vi "Main.vi"() -> ()   [LabVIEW 2018]
uses:
  ctl/State.ctl
panel:
  out "시간계산":i32
  out "조리 시간":string
  in  "10초":bool
  in  "30초":bool
  in  "1분":bool
  in  "정지":bool
  out "출력 메세지":string
  in  "문 열림":bool
  in  "조리 시작":bool
  # "전자레인지"
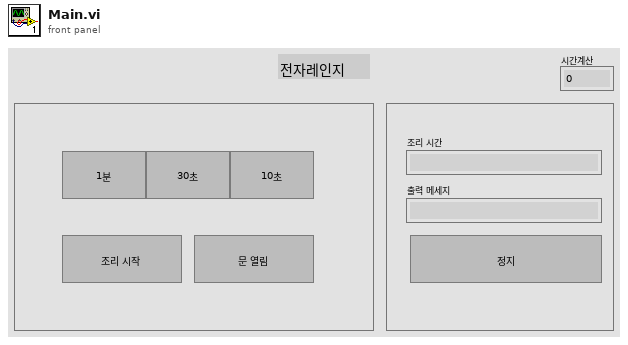
[diagram p1: front panel]
types:
  T1 = typedef "State.ctl" = enum16{"대기", "조리", "문열림", "조리완료", "일시정지"}
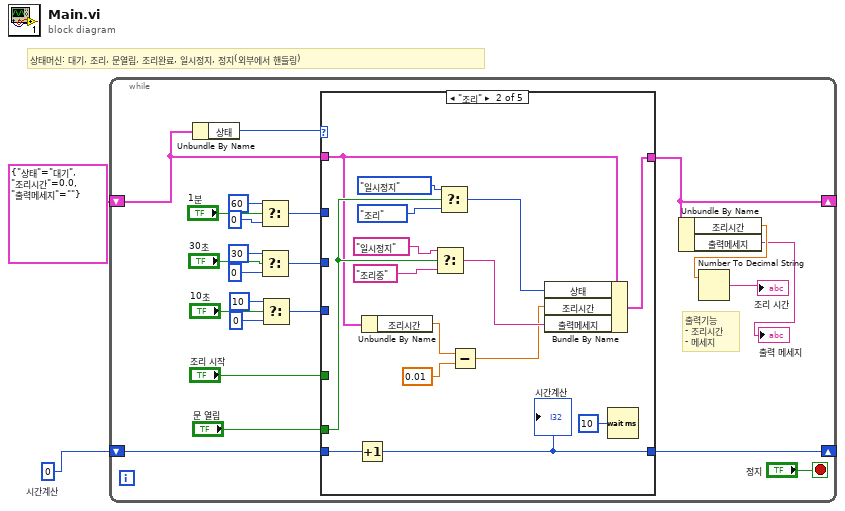
[diagram p0: block diagram]
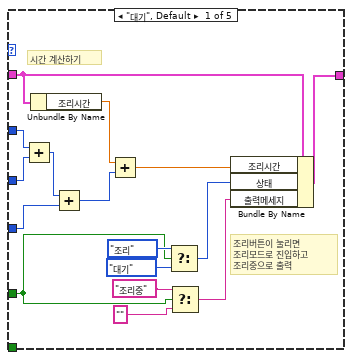
[diagram p2: hidden frame]
diagram:
  w1 = 0  # 시간계산
  # "상태머신: 대기, 조리, 문열림, 조리완료, 일시정지, 정지(외부에서 핸들링)"
  n1 = while {
    shift-right: [w9] -> _
    shift-left: cluster{"상태":T1, "조리시간":dbl, "출력메세지":string} {"상태"=enum."대기", "조리시간"=0.0, "출력메세지"=""} -> [w25]
    shift-right: [w4] -> _
    shift-left: w1 -> [w5]
    stop <- "정지" stop-if-true
    # "출력기능\n- 조리시간\n- 메세지"
    n2 = Unbundle By Name(w25) -> ("상태"=w14:T1)
    n3 = Select(t=60, s="1분", f=0) -> (s? t:f=w13:i32)
    n4 = Select(t=30, s="30초", f=0) -> (s? t:f=w12:i32)
    n5 = Select(t=10, s="10초", f=0) -> (s? t:f=w11:i32)
    n6 = case shown="\"조리\"" w14 {
      tunnel: w25 -> [w35 w45 _ _ w57]
      tunnel: w13 -> [w41 _ _ _ _]
      tunnel: w12 -> [w40 _ _ _ _]
      tunnel: w11 -> [w39 _ _ _ _]
      tunnel: [w33 w46 _ _ w57] -> w9
      tunnel: "조리 시작" -> [w27 _ _ _ _]
      tunnel: w5 -> [_ w56 _ _ _]
      tunnel: [_ w55 _ _ _] -> w4
      tunnel: "문 열림" -> [_ w50 _ _ _]
      frame "대기", Default {
        # "조리버튼이 눌리면\n조리모드로 진입하고\n조리중으로 출력"
        # "시간 계산하기"
        n7 = Add(x=w41, y=w40) -> (x+y=w38:i32)
        n8 = Unbundle By Name(w35) -> ("조리시간"=w37:dbl)
        n9 = Add(x=w38, y=w39) -> (x+y=w36:i32)
        n10 = Add(x=w37, y=w36) -> (x+y=w34:dbl)
        n11 = Select(t=State."조리" ("상태 2"), s=w27, f=State."대기" ("상태 2")) -> (s? t:f=w30:T1)
        n12 = Select(t="조리중", s=w27, f="") -> (s? t:f=w26:string)
        n13 = Bundle By Name ("이름으로 묶기")(cluster=w35, "조리시간"=w34, "상태"=w30, "출력메세지"=w26) -> (w33:cluster{"상태":T1, "조리시간":dbl, "출력메세지":string})
      }
      frame "조리" {
        n14 = Increment(x=w56) -> (x+1=w55:i32)
        "시간계산" <- w55
        n15 = Unbundle By Name(w45) -> ("조리시간"=w44:dbl)
        n16 = Select(t="일시정지", s=w50, f="조리중") -> (s? t:f=w47:string)
        n17 = Select(t=State."일시정지" ("상태 2"), s=w50, f=State."조리" ("상태 2")) -> (s? t:f=w51:T1)
        n18 = Subtract(x=w44, y=0.01) -> (x-y=w42:dbl)
        n19 = Bundle By Name(cluster=w45, "상태"=w51, "조리시간"=w42, "출력메세지"=w47) -> (w46:cluster{"상태":T1, "조리시간":dbl, "출력메세지":string})
        n20 = Wait (ms)(milliseconds to wait=u32 10 ("대기 시간 (ms)")) -> ()  [unwired: 1 out]
      }
      frame "문열림" {
      }
      frame "조리완료" {
      }
      frame "일시정지" {
      }
    }
    n21 = Unbundle By Name(w9) -> ("조리시간"=w8:dbl, "출력메세지"=→"출력 메세지":string)
    n22 = Number To Decimal String(number=w8) -> (decimal integer string=→"조리 시간":string)  [unwired: 1 in]
  }
